vi "gantry vs OGP test.vi"() -> ()   [LabVIEW 2021]
uses:
  Program Files (x86)/National Instruments/LabVIEW 2021/examples/Connectivity/Python/support/PythonVersionsEnum.ctl
  <vilib>/Utility/file.llb/Read Delimited Spreadsheet (DBL).vi
panel:
  out "Array":dbl[][][](array[numeric])
  out "Pos2 rotation":dbl
  out "Pos1 rotation":dbl
  out "Pos2 Offset":dbl[](array[numeric])
  out "Pos2 Center":dbl[](array[numeric])
  out "Pos1 Offset":dbl[](array[numeric])
  out "Pos1 center":dbl[](array[numeric])
  out "F2":dbl[](array[numeric])
  out "F1":dbl[](array[numeric])
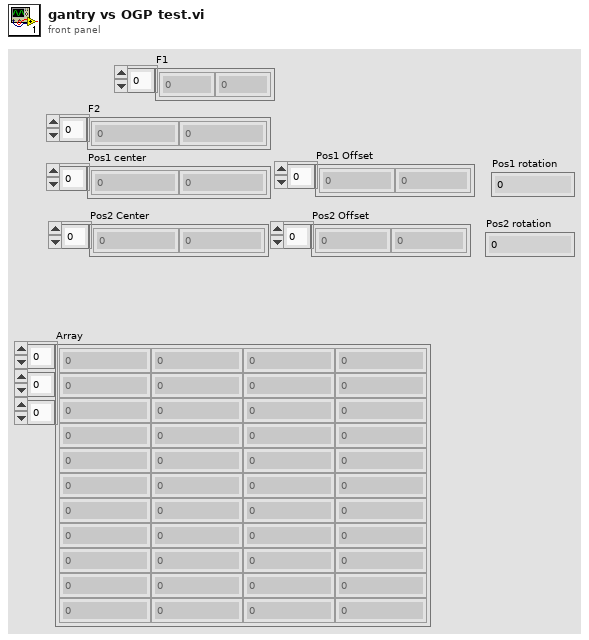
[diagram p1: front panel]
types:
  T1 = typedef "File Paths.ctl" = cluster{"Glue Pattern Folder":path, "Carrier Tray Folder":path, "Pick Up Tool Fixture Folder":path, "Components Folder":path, "Bellows Tool Offset.txt":path, "Pick Up Tool Offset.txt":path, "Dispense Tip Offset.txt":path, "Log Files":path, "Gantry Assembly Map.txt":path, "Syringe and offset map.txt":path}
  T2 = typedef "PythonVersionsEnum.ctl" = enum16{"3.6", "3.7", "3.8", "3.9"}
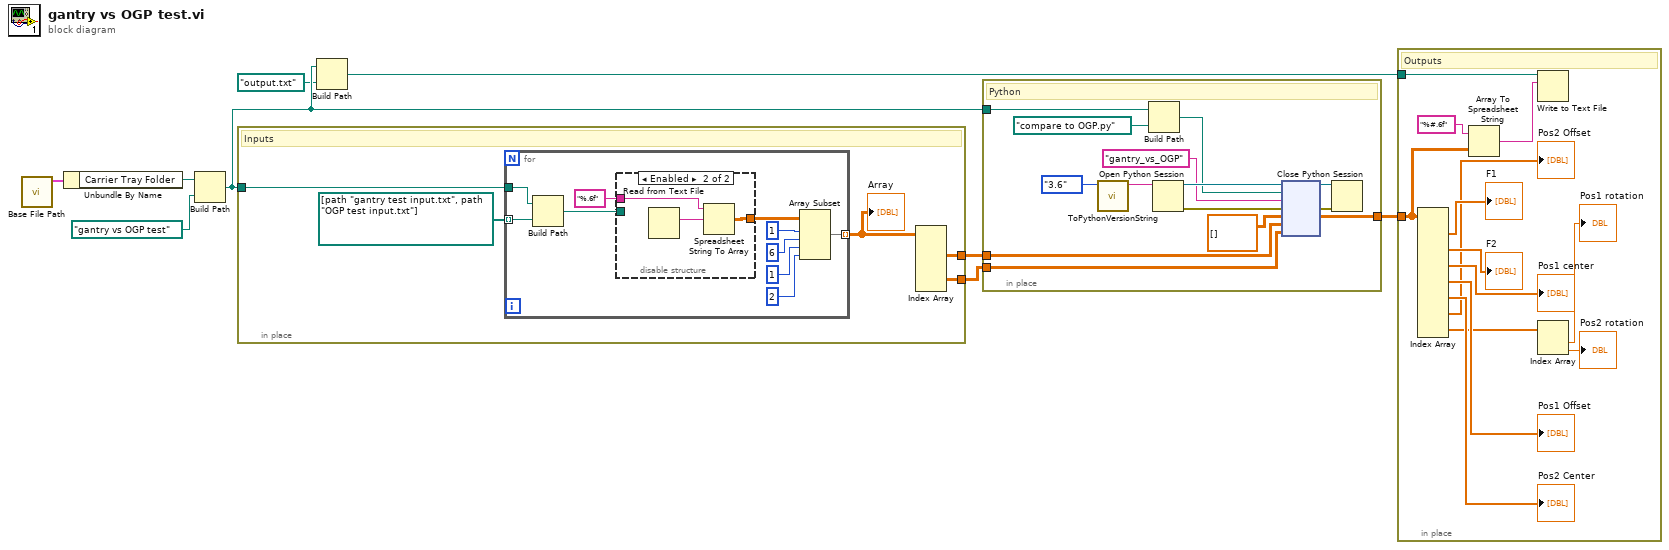
[diagram p0: block diagram]
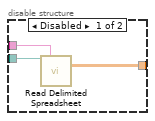
[diagram p2: hidden frame]
diagram:
  n1 = call "Base File Path.vi"() -> ("Paths Out"=w6:T1)  [unwired: 11 in]
  n2 = Unbundle By Name(w6) -> ("Carrier Tray Folder"=w5:path)
  n3 = Build Path(base path=w5, name or relative path=path "gantry vs OGP test") -> (appended path=w2:path)
  n4 = in-place {
    in-place-border: [w12] -> w9
    in-place-border: [w11] -> w8
    in-place-border: w2 -> [w10]
    # "Inputs"
    n5 = for {
      tunnel: [w18] -> w13 mode=indexing
      tunnel: path[] [path "gantry test input.txt", path "OGP test input.txt"] ("name or relative path") -> [w16] mode=indexing
      tunnel: w10 -> [w15]
      n6 = Build Path(base path=w15, name or relative path=w16) -> (appended path=w17:path)
      n7 = disable-structure shown="Enabled" {
        disable-tunnel: "%.6f" ("format (%.3f)") -> [w27 w29]
        disable-tunnel: [w26 w28] -> w23
        disable-tunnel: w17 -> [w25 _]
        frame Disabled {
          n8 = call-poly <vilib>:"Read Delimited Spreadsheet.vi"("file path (dialog if empty)"=w25, "format (%.3f)"=w27) -> ("all rows"=w26:dbl[][])  [unwired: 8 in, 5 out]
        }
        frame Enabled {
          n9 = Read from Text File() -> (text=w30:string)  [unwired: 4 in, 3 out]
          n10 = Spreadsheet String To Array(format string=w29, spreadsheet string=w30) -> (array=w28:dbl[][])  [unwired: 2 in]
        }
      }
      n11 = Array Subset(array=w23, index (row)=1 ("index"), length (row)=6 ("length"), index (col)=1 ("index"), length (col)=2 ("length")) -> (w18:dbl[][])
    }
    "Array" <- w13
    n12 = Index Array(array=w13) -> (element #1=w12:dbl[][], element #2=w11:dbl[][])  [unwired: 6 in]
  }
  n13 = Build Path(base path=w2, name or relative path=path "output.txt") -> (appended path=w3:path)
  n14 = in-place {
    in-place-border: w9 -> [w44]
    in-place-border: w8 -> [w43]
    in-place-border: [w32] -> w7
    in-place-border: w2 -> [w31]
    # "Python"
    n15 = call "ToPythonVersionString.vi"("python version"=PythonVersionsEnum."3.6") -> ("python version string"=w41:string)  [unwired: 10 in]
    n16 = Build Path(base path=w31, name or relative path=path "compare to OGP.py") -> (appended path=w34:path)
    n17 = Open Python Session(python version=w41) -> (session out=w40:refnum<k35>, error out=w38:errorcluster)  [unwired: 2 in]
    n18 = node(w40, w34, "gantry_vs_OGP" ("function name"), w38, dbl[][] [], w44, w43) -> (w39:refnum<k35>, w37:errorcluster, w32:dbl[][])  [unwired: 2 in, 2 out]
    n19 = Close Python Session(session in=w39, error in=w37) -> ()  [unwired: 1 out]
  }
  n20 = in-place {
    in-place-border: w7 -> [w46]
    in-place-border: w3 -> [w45]
    # "Outputs"
    n21 = Index Array(array=w46) -> (element #1=→"F1":dbl[], element #2=→"F2":dbl[], element #3=→"Pos1 center":dbl[], element #4=→"Pos1 Offset":dbl[], element #5=→"Pos2 Center":dbl[], element #6=→"Pos2 Offset":dbl[], element #7=w51:dbl[])  [unwired: 14 in]
    n22 = Array To Spreadsheet String(array=w46, 3:"%#.6f" ("format string")) -> (spreadsheet string=w48:string)  [unwired: 1 in]
    n23 = Write to Text File(file (use dialog)=w45, text=w48) -> ()  [unwired: 2 in, 3 out]
    n24 = Index Array(array=w51) -> (element #1=→"Pos1 rotation":dbl, element #2=→"Pos2 rotation":dbl)  [unwired: 2 in]
  }
